vi "Write_camera_csv.vi"(10 "Image Pixels (U16)":u16[][](array[numeric]), 11 "seconds\n between acquistions":u32) -> ()   [LabVIEW 2023]
uses:
  <vilib>/Utility/file.llb/Write Delimited Spreadsheet (I64).vi
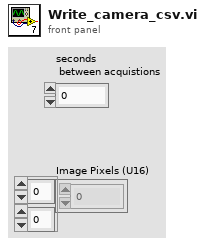
[diagram p1: front panel]
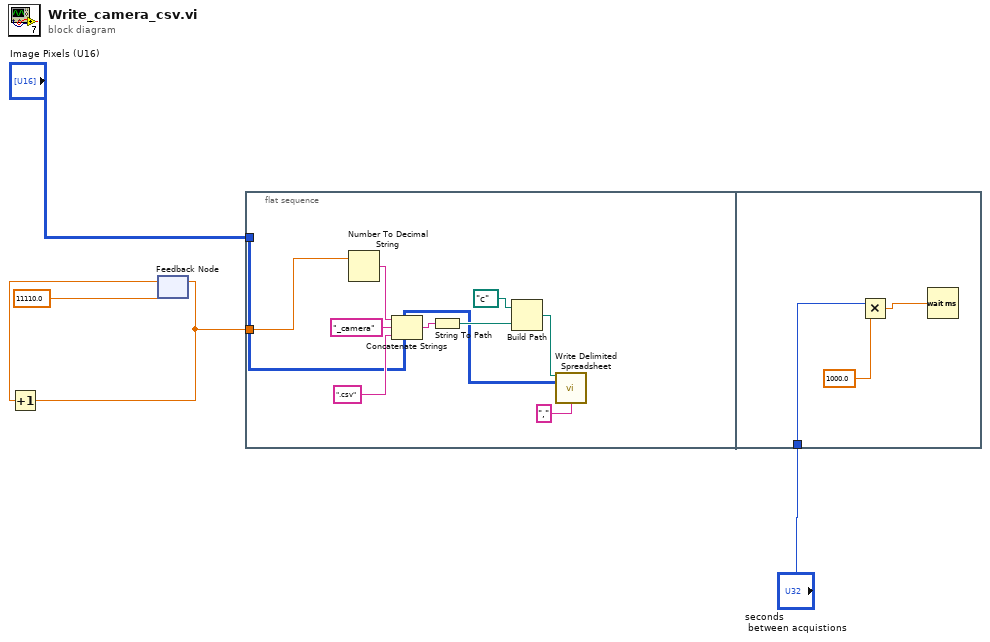
[diagram p0: block diagram]
diagram:
  n1 = feedback #1(11110.0) -> (w3:dbl)
  n2 = Increment(x=w3) -> (x+1=w4:dbl)
  n3 = feedback-in #1(w4) -> ()
  n4 = flat-sequence {
    tunnel: w4 -> [w10]
    tunnel: "Image Pixels (U16)" -> [w6]
    tunnel: "seconds\n between acquistions" -> [w16]
    frame #0 {
      n5 = Number To Decimal String(number=w10) -> (decimal integer string=w14:string)  [unwired: 1 in]
      n6 = Concatenate Strings(w14, "_camera" ("string"), ".csv" ("string")) -> (w15:string)
      n7 = String To Path(string=w15) -> (path=w13:path)
      n8 = Build Path(base path=path "c:/", name or relative path=w13) -> (appended path=w12:path)
      n9 = call-poly <vilib>:"Write Delimited Spreadsheet.vi"("file path (dialog if empty)"=w12, "2D data"=w6, "delimiter (\\t)"="," ("delimiter (\\t)")) -> ()  [unwired: 11 in, 2 out]
    }
    frame #1 {
      n10 = Multiply(x=w16, y=1000.0) -> (x*y=w17:dbl)
      n11 = Wait (ms)(milliseconds to wait=w17) -> ()  [unwired: 1 out]
    }
  }
